vi "hardware_close_hardware.vi"(8 "error in (no error)":errorcluster, 11 "hydraharp in":refnum<class "picoharp.lvclass">) -> (0 "error out":errorcluster, 3 "hydraharp out":refnum<class "picoharp.lvclass">)   [LabVIEW 2015, in "picoharp.lvclass"]
uses:
  picoharp.lvclass
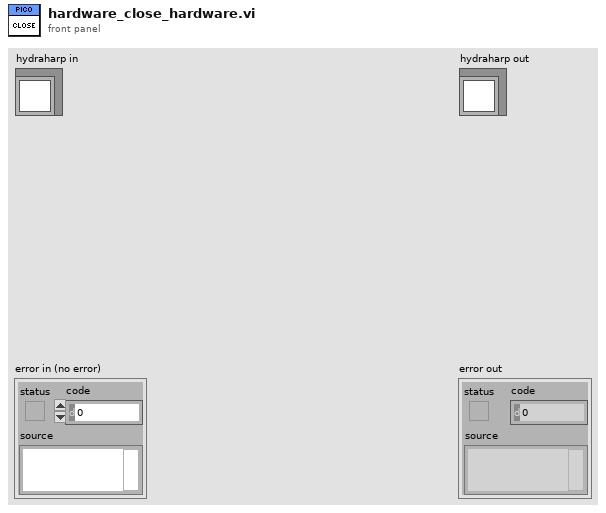
[diagram p1: front panel]
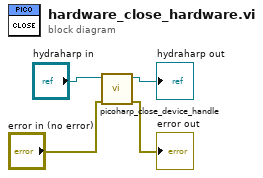
[diagram p0: block diagram]
diagram:
  n1 = call "picoharp_close_device_handle.vi"("error in (no error)"="error in (no error)", "hydraharp in"="hydraharp in") -> ("error out"=→"error out":errorcluster, "hydraharp out"=→"hydraharp out":refnum<class "picoharp.lvclass">)  [unwired: 8 in]
